vi "Write Graph to excel.vi"(8 "error in (no error)":errorcluster, 11 "Graph":refnum<vi>) -> (0 "error out":errorcluster, 2 "excel data":string[][](array[string]))   [LabVIEW 2020]
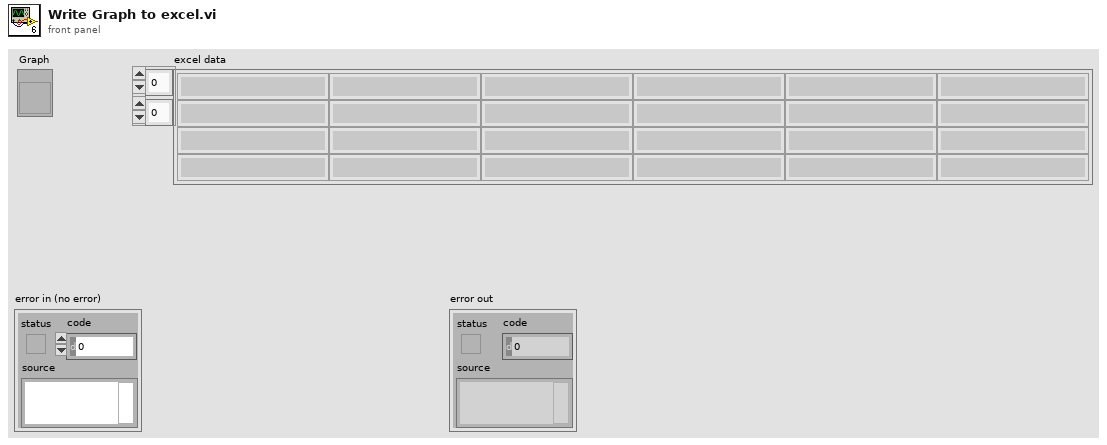
[diagram p1: front panel]
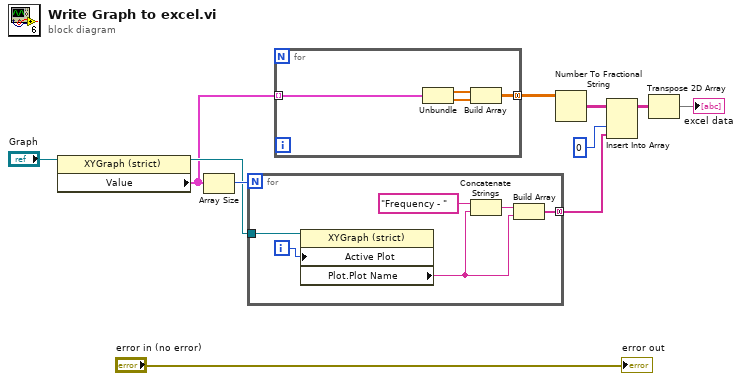
[diagram p0: block diagram]
diagram:
  n1 = property class="XYGraph (strict)"(reference="Graph") -> (reference out=w3:refnum<vi>, "Value"=w2:cluster{"频率":dbl[], dbl[]}[])  [unwired: 1 in, 1 out]
  n2 = Array Size(array=w2) -> (size(s)=w11:i32)
  n3 = for {
    N: w11 -> [_]
    tunnel: [w15] -> w7 mode=concatenating
    tunnel: w3 -> [w14]
    i -> [w13]
    n4 = property class="XYGraph (strict)"(reference=w14, "Active Plot"=w13) -> ("Plot.Plot Name"=w12:string)  [unwired: 1 in, 2 out]
    n5 = Concatenate Strings("Frequency - ", w12) -> (w16:string)
    n6 = Build Array(w16, w12) -> (w15:string[])
  }
  n7 = for {
    tunnel: w2 -> [w20] mode=indexing
    tunnel: [w21] -> w10 mode=concatenating
    n8 = Unbundle(w20) -> ("频率"=w19:dbl[], w18:dbl[])
    n9 = Build Array(w19, w18) -> (w21:dbl[][])
  }
  n10 = Number To Fractional String(number=w10) -> (F-format string=w9:string[][])  [unwired: 3 in]
  n11 = Insert Into Array(array=w9, index (col)=0 ("disabled index (col)"), new element=w7) -> (w6:string[][])  [unwired: 1 in]
  n12 = Transpose 2D Array(2D array=w6) -> (transposed array=→"excel data":string[][])
  "error out" <- "error in (no error)"
